vi "CMC_Homework_07.vi"() -> ()   [LabVIEW 2013]
panel:
  in  "STOP COUNTING":bool
  in  "DISPLAY COUNTS":bool
  out "COLOR COUNTER":T1={"RED"=11, "BLUE"=12, "GREEN"=19, "YELLOW"=9, "BROWN"=22, "ORANGE"=15} {"ORANGE" scale=0.0..100.0; "BROWN" scale=0.0..100.0; "YELLOW" scale=0.0..100.0; "GREEN" scale=0.0..100.0; "BLUE" scale=0.0..100.0; "RED" scale=0.0..100.0}
  # "Created in collaboration with Sarah Bailey"
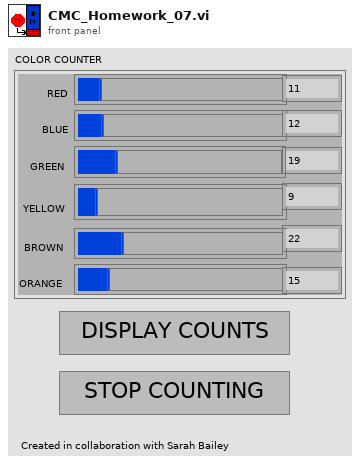
[diagram p1: front panel]
types:
  T1 = cluster{"RED":u8, "BLUE":u8, "GREEN":u8, "YELLOW":u8, "BROWN":u8, "ORANGE":u8}
  T2 = enum16{"Left Button", "Center Button", "Right Button", "Window Close"}
  T3 = enum16{"Red", "Blue", "Green", "Yellow", "Brown", "Orange"}
  T4 = cluster{"Cluster[0]":u8, "Cluster[1]":u8, "Cluster[2]":u8, "Cluster[3]":u8, "Cluster[4]":u8, "Cluster[5]":u8}
  T5 = cluster{"Value[0]":u8, "Value[1]":u8, "Value[2]":u8, "Value[3]":u8, "Value[4]":u8, "Value[5]":u8}
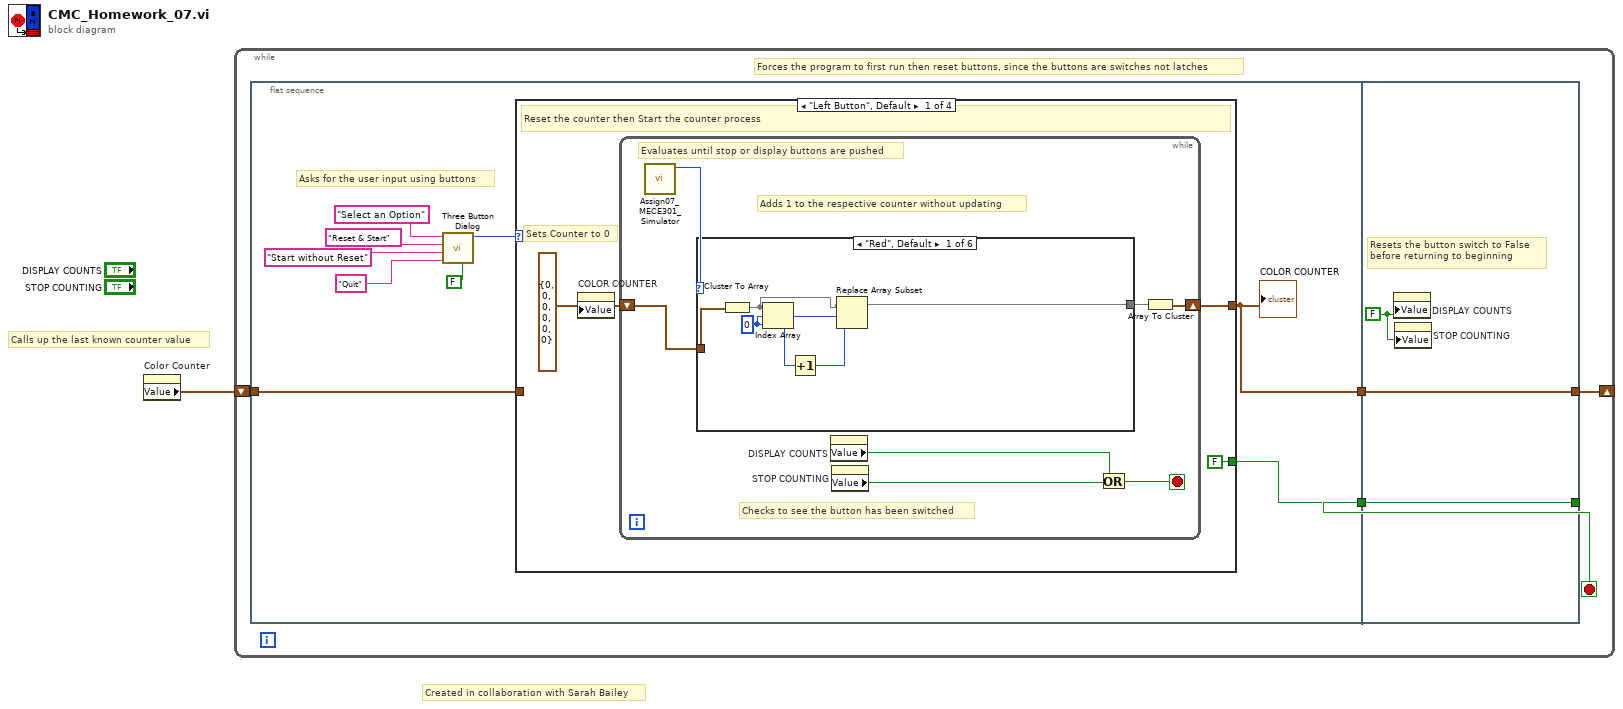
[diagram p0: block diagram]
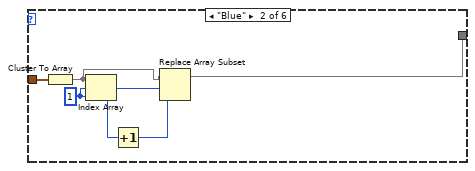
[diagram p2: hidden frame]
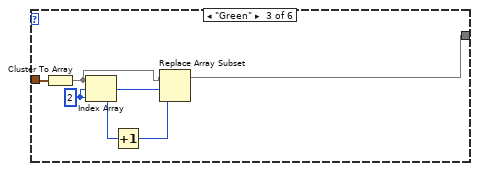
[diagram p3: hidden frame]
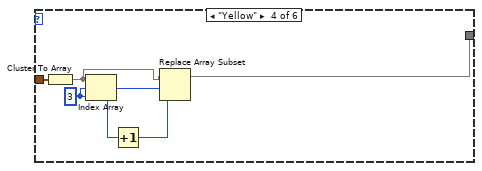
[diagram p4: hidden frame]
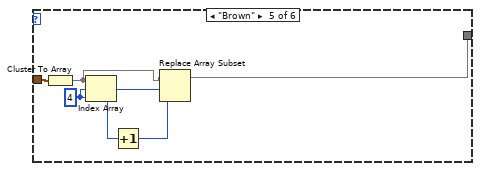
[diagram p5: hidden frame]
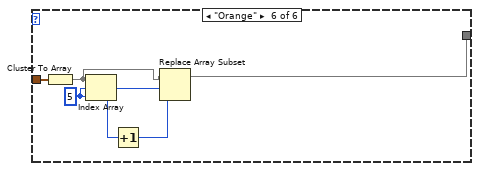
[diagram p6: hidden frame]
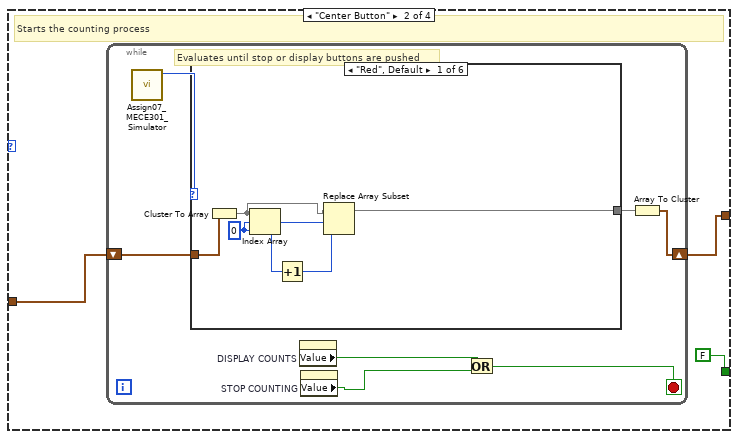
[diagram p7: hidden frame]
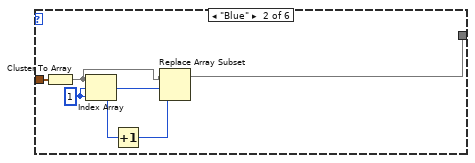
[diagram p8: hidden frame]
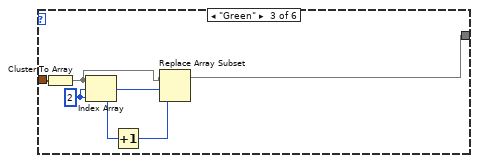
[diagram p9: hidden frame]
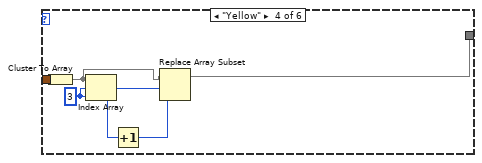
[diagram p10: hidden frame]
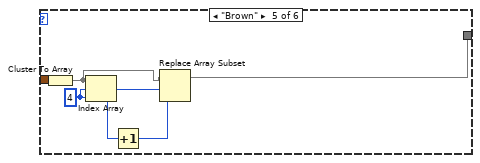
[diagram p11: hidden frame]
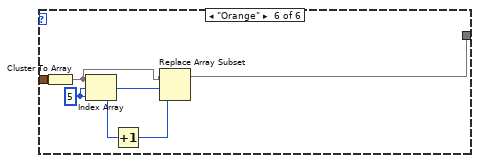
[diagram p12: hidden frame]
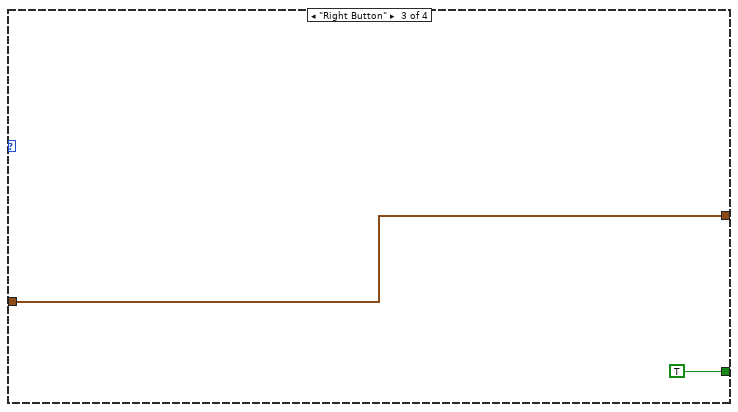
[diagram p13: hidden frame]
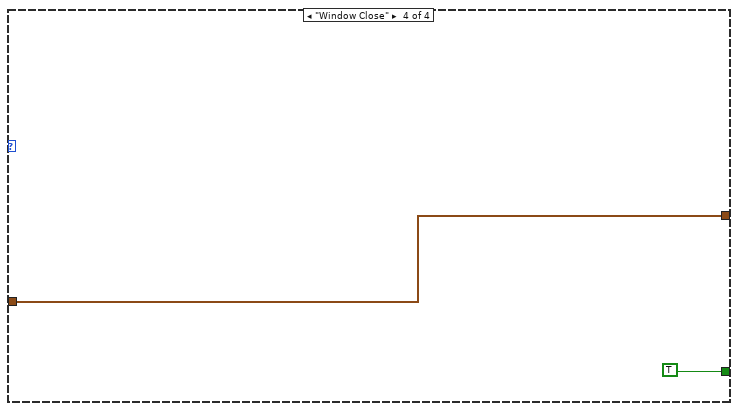
[diagram p14: hidden frame]
diagram:
  # "Created in collaboration with Sarah Bailey"
  # "Calls up the last known counter value"
  n1 = property on="Color Counter" class="Clust (strict)"() -> ("Value"=w1:T1)  [unwired: 2 in, 2 out]
  n2 = while {
    shift-right: [w5] -> _
    shift-left: w1 -> [w6]
    stop <- w4 stop-if-true
    # "Forces the program to first run then reset buttons, since the buttons are switches not latches"
    n3 = flat-sequence {
      tunnel: w6 -> [w9]
      tunnel: [w8] -> w3
      tunnel: [w7] -> w2
      tunnel: [w113] -> w4
      tunnel: [w114] -> w5
      tunnel: w3 -> [w114]
      tunnel: w2 -> [w113]
      frame #0 {
        # "Asks for the user input using buttons"
        n4 = call <vilib>:"Three Button Dialog.vi"("Allow user to close window? (TRUE)"=FALSE, "Right Button Text (\"Cancel\")"="Quit" ("Right Button Text (\"Cancel\")"), "Center Button Text (\"No\")"="Start without Reset" ("Center Button Text (\"No\")"), "Left Button Text (\"Yes\")"="Reset & Start" ("Left Button Text (\"Yes\")"), "message"="Select an Option") -> ("Which Button?"=w15:T2)  [unwired: 6 in]
        n5 = case shown="\"Left Button\", Default" w15 {
          tunnel: w9 -> [_ w64 w109 w111]
          tunnel: [w16 w63 w109 w111] -> w8
          tunnel: [FALSE FALSE TRUE TRUE] -> w7
          frame "Left Button", Default {
            w18 = T1 {"RED"=0, "BLUE"=0, "GREEN"=0, "YELLOW"=0, "BROWN"=0, "ORANGE"=0} ("Cluster")
            # "Sets Counter to 0"
            # "Reset the counter then Start the counter process"
            n6 = property on="COLOR COUNTER" class="Clust (strict)"("Value"=w18) -> ()  [unwired: 2 in, 2 out]
            n7 = while {
              shift-right: [w19] -> w16
              shift-left: w18 -> [w24]
              stop <- w22 stop-if-true
              # "Checks to see the button has been switched"
              # "Adds 1 to the respective counter without updating"
              # "Evaluates until stop or display buttons are pushed"
              n8 = call "Assign07_MECE301_Simulator.vi"() -> ("Color"=w25:T3)  [unwired: 11 in]
              n9 = case shown="\"Red\", Default" w25 {
                tunnel: w24 -> [w31 w33 w39 w45 w51 w57]
                tunnel: [w26 w32 w38 w44 w50 w56] -> w23
                frame "Red", Default {
                  w27 = 0 ("index")
                  n10 = Cluster To Array(cluster=w31) -> (array=w28:u8[])
                  n11 = Index Array(array=w28, index=w27) -> (element=w30:u8)
                  n12 = Increment(x=w30) -> (x+1=w29:u8)
                  n13 = Replace Array Subset(array=w28, new element=w29, index=w27) -> (w26:u8[])
                }
                frame "Blue" {
                  w34 = 1 ("index")
                  n14 = Cluster To Array(cluster=w33) -> (array=w35:u8[])
                  n15 = Index Array(array=w35, index=w34) -> (element=w37:u8)
                  n16 = Increment(x=w37) -> (x+1=w36:u8)
                  n17 = Replace Array Subset(array=w35, new element=w36, index=w34) -> (w32:u8[])
                }
                frame "Green" {
                  w40 = 2 ("index")
                  n18 = Cluster To Array(cluster=w39) -> (array=w41:u8[])
                  n19 = Index Array(array=w41, index=w40) -> (element=w43:u8)
                  n20 = Increment(x=w43) -> (x+1=w42:u8)
                  n21 = Replace Array Subset(array=w41, new element=w42, index=w40) -> (w38:u8[])
                }
                frame "Yellow" {
                  w46 = 3 ("index")
                  n22 = Cluster To Array(cluster=w45) -> (array=w47:u8[])
                  n23 = Index Array(array=w47, index=w46) -> (element=w49:u8)
                  n24 = Increment(x=w49) -> (x+1=w48:u8)
                  n25 = Replace Array Subset(array=w47, new element=w48, index=w46) -> (w44:u8[])
                }
                frame "Brown" {
                  w52 = 4 ("index")
                  n26 = Cluster To Array(cluster=w51) -> (array=w53:u8[])
                  n27 = Index Array(array=w53, index=w52) -> (element=w55:u8)
                  n28 = Increment(x=w55) -> (x+1=w54:u8)
                  n29 = Replace Array Subset(array=w53, new element=w54, index=w52) -> (w50:u8[])
                }
                frame "Orange" {
                  w58 = 5 ("index")
                  n30 = Cluster To Array(cluster=w57) -> (array=w59:u8[])
                  n31 = Index Array(array=w59, index=w58) -> (element=w61:u8)
                  n32 = Increment(x=w61) -> (x+1=w60:u8)
                  n33 = Replace Array Subset(array=w59, new element=w60, index=w58) -> (w56:u8[])
                }
              }
              n34 = property on="DISPLAY COUNTS" class="Bool (strict)"() -> ("Value"=w21:bool)  [unwired: 2 in, 2 out]
              n35 = property on="STOP COUNTING" class="Bool (strict)"() -> ("Value"=w20:bool)  [unwired: 2 in, 2 out]
              n36 = Or(x=w21, y=w20) -> (x .or. y?=w22:bool)
              n37 = Array To Cluster(array=w23) -> (cluster=w19:T4)
            }
          }
          frame "Center Button" {
            # "Starts the counting process"
            n38 = while {
              shift-right: [w68] -> w63
              shift-left: w64 -> [w70]
              stop <- w67 stop-if-true
              # "Evaluates until stop or display buttons are pushed"
              n39 = call "Assign07_MECE301_Simulator.vi"() -> ("Color"=w71:T3)  [unwired: 11 in]
              n40 = case shown="\"Red\", Default" w71 {
                tunnel: w70 -> [w72 w79 w85 w91 w97 w103]
                tunnel: [w73 w78 w84 w90 w96 w102] -> w69
                frame "Red", Default {
                  w74 = 0 ("index")
                  n41 = Cluster To Array(cluster=w72) -> (array=w75:u8[])
                  n42 = Index Array(array=w75, index=w74) -> (element=w77:u8)
                  n43 = Increment(x=w77) -> (x+1=w76:u8)
                  n44 = Replace Array Subset(array=w75, new element=w76, index=w74) -> (w73:u8[])
                }
                frame "Blue" {
                  w80 = 1 ("index")
                  n45 = Cluster To Array(cluster=w79) -> (array=w81:u8[])
                  n46 = Index Array(array=w81, index=w80) -> (element=w83:u8)
                  n47 = Increment(x=w83) -> (x+1=w82:u8)
                  n48 = Replace Array Subset(array=w81, new element=w82, index=w80) -> (w78:u8[])
                }
                frame "Green" {
                  w86 = 2 ("index")
                  n49 = Cluster To Array(cluster=w85) -> (array=w87:u8[])
                  n50 = Index Array(array=w87, index=w86) -> (element=w89:u8)
                  n51 = Increment(x=w89) -> (x+1=w88:u8)
                  n52 = Replace Array Subset(array=w87, new element=w88, index=w86) -> (w84:u8[])
                }
                frame "Yellow" {
                  w92 = 3 ("index")
                  n53 = Cluster To Array(cluster=w91) -> (array=w93:u8[])
                  n54 = Index Array(array=w93, index=w92) -> (element=w95:u8)
                  n55 = Increment(x=w95) -> (x+1=w94:u8)
                  n56 = Replace Array Subset(array=w93, new element=w94, index=w92) -> (w90:u8[])
                }
                frame "Brown" {
                  w98 = 4 ("index")
                  n57 = Cluster To Array(cluster=w97) -> (array=w99:u8[])
                  n58 = Index Array(array=w99, index=w98) -> (element=w101:u8)
                  n59 = Increment(x=w101) -> (x+1=w100:u8)
                  n60 = Replace Array Subset(array=w99, new element=w100, index=w98) -> (w96:u8[])
                }
                frame "Orange" {
                  w104 = 5 ("index")
                  n61 = Cluster To Array(cluster=w103) -> (array=w105:u8[])
                  n62 = Index Array(array=w105, index=w104) -> (element=w107:u8)
                  n63 = Increment(x=w107) -> (x+1=w106:u8)
                  n64 = Replace Array Subset(array=w105, new element=w106, index=w104) -> (w102:u8[])
                }
              }
              n65 = property on="DISPLAY COUNTS" class="Bool (strict)"() -> ("Value"=w66:bool)  [unwired: 2 in, 2 out]
              n66 = property on="STOP COUNTING" class="Bool (strict)"() -> ("Value"=w65:bool)  [unwired: 2 in, 2 out]
              n67 = Or(x=w66, y=w65) -> (x .or. y?=w67:bool)
              n68 = Array To Cluster(array=w69) -> (cluster=w68:T5)
            }
          }
          frame "Right Button" {
          }
          frame "Window Close" {
          }
        }
        "COLOR COUNTER" <- w8
      }
      frame #1 {
        w112 = FALSE
        # "Resets the button switch to False \nbefore returning to beginning"
        n69 = property on="DISPLAY COUNTS" class="Bool (strict)"("Value"=w112) -> ()  [unwired: 2 in, 2 out]
        n70 = property on="STOP COUNTING" class="Bool (strict)"("Value"=w112) -> ()  [unwired: 2 in, 2 out]
      }
    }
  }
